vi "Initialize and Register Sessions.vi"(8 "error in":errorcluster, 11 "sequence context in":refnum<k7>) -> (0 "error out":errorcluster)   [LabVIEW 2021, in "SourceMeasureDCVoltage.lvlib"]
uses:
  SourceMeasureDCVoltage.lvlib
  <vilib>/gRPC/Generated APIs/ni/measurementlink/sessionmanagement/v1/RPC Messages/ni_measurementlink_PinMapContext.ctl
  <vilib>/Plug-In SDKs/Clients/Session Management V1/Session Reservation/Session Reservation.lvclass/Session Reservation.ctl
  FAL/Instruments/Abstract_Instrument/controls/Initialize_Info.ctl
  <vilib>/Plug-In SDKs/Clients/Session Management V1/Session Reservation/Initialize and Close Session Behavior.ctl
  <vilib>/Plug-In SDKs/Clients/Session Management V1/Session Reservation/Merge Invalid DVR Error.vi
  <vilib>/Plug-In SDKs/Clients/Session Management V1/Session Reservation/Is DVR Valid.vi
  <vilib>/Plug-In SDKs/Measurements/Helpers/Error Strings Global Internal.vi
  <vilib>/Utility/error.llb/Error Cluster From Error Code.vi
  FAL/Instruments/Abstract_Instrument/Abstract_Instrument.lvclass
  <vilib>/Plug-In SDKs/Clients/Session Management V1/Session Reservation/Session Reservation.lvclass
  <vilib>/Plug-In SDKs/TestStand/NI Pin Map TestStand.lvlib
  <vilib>/gRPC/Generated APIs/ni/measurementlink/sessionmanagement/v1/ni.measurementlink.sessionmanagement.v1.api.lvlib
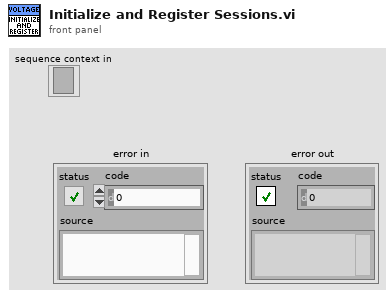
[diagram p1: front panel]
types:
  T1 = typedef "ni.measurementlink.sessionmanagement.v1.api.lvlib/ni_measurementlink_PinMapContext.ctl" = cluster{"pin_map_id":string, "sites":i32[]}
  T2 = typedef "Abstract_Instrument.lvclass/Initialize_Info.ctl" = cluster{"initialize and close session behavior":T3, "reset":bool, "optional string":string}
  T3 = typedef "NI Session Management V1 Client.lvlib/Session Reservation.lvclass/Initialize and Close Session Behavior.ctl" = enum16{"Auto", "Initialize and Close", "Attach and Detach", "Initialize and Detach", "Attach and Close"}
  T4 = typedef "ni.measurementlink.sessionmanagement.v1.api.lvlib/ni_measurementlink_sessionmanagement_v1_SessionInformation.ctl" = cluster{"session":T5, "resource_name":string, "channel_list":string, "instrument_type_id":string, "session_exists":bool, "channel_mappings":T6[]}
  T5 = typedef "ni.measurementlink.sessionmanagement.v1.api.lvlib/nidevice_grpc_Session.ctl" = cluster{"name":string}
  T6 = typedef "ni.measurementlink.sessionmanagement.v1.api.lvlib/ni_measurementlink_sessionmanagement_v1_ChannelMapping.ctl" = cluster{"pin_or_relay_name":string, "site":i32, "channel":string, "multiplexer_resource_name":string, "multiplexer_route":string}
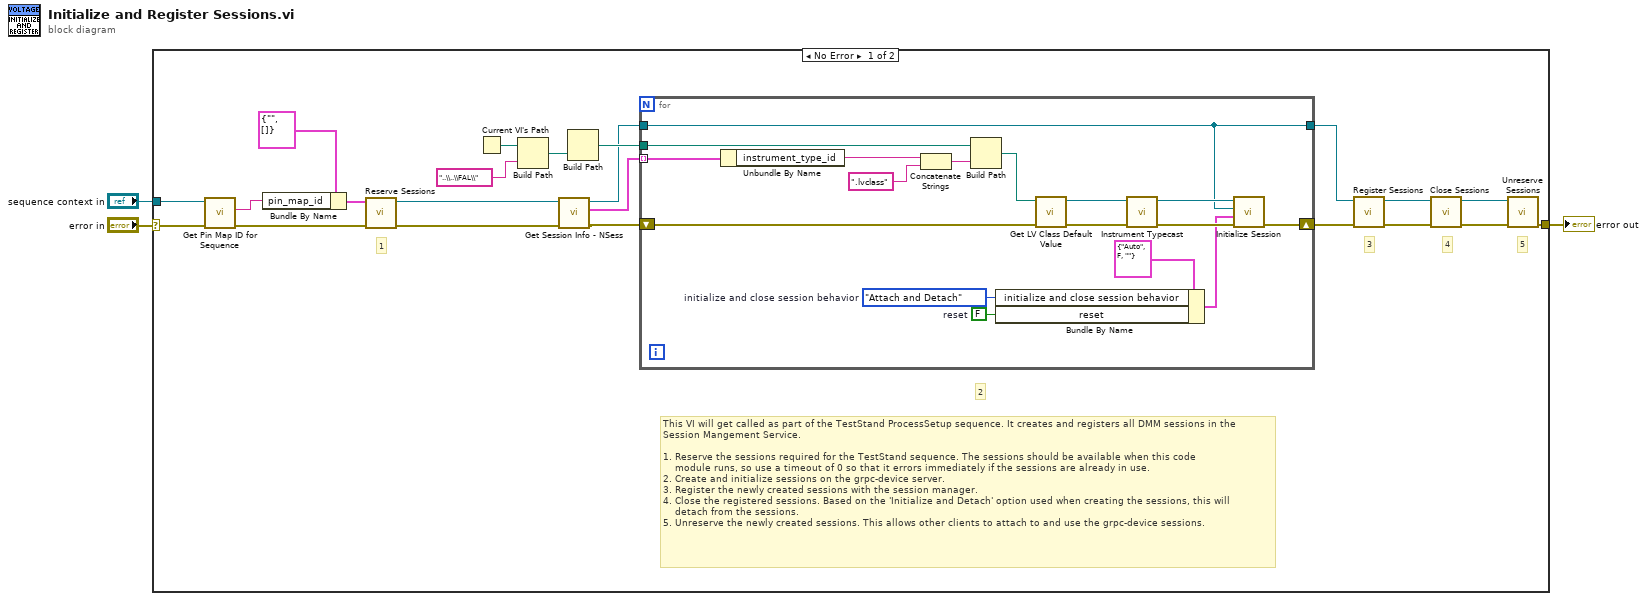
[diagram p0: block diagram]
diagram:
  n1 = case shown="No Error" "error in" {
    selector: "error in" -> [w24 w43]
    tunnel: "sequence context in" -> [w25 _]
    tunnel: [w6 w43] -> w1
    frame No Error {
      # "5"
      # "4"
      # "3"
      # "2"
      # "1"
      # "This VI will get called as part of the TestStand ProcessSetup sequence. It creates and registers all DMM sessions in the\nSession Mangement Service.\n\n1. Reserve the sessions required for the TestStand sequence. The sessions should be available when this code\n    module runs, so use a timeout of 0 so that it errors immediately if the sessions are already in use.  \n2. Create and initialize sessions on the grpc-device server.\n3. Register the newly created sessions with the session manager.\n4. Close the registered sessions. Based on the 'Initialize and Detach' option used when creating the sessions, this will\n    detach from the sessions.\n5. Unreserve the newly created sessions. This allows other clients to attach to and use the grpc-device sessions."
      n2 = call <vilib>:"Get Pin Map ID for Sequence.vi"("error in"=w24, "sequence context in"=w25) -> ("error out"=w23:errorcluster, "pin map id"=w22:string)  [unwired: 7 in, 1 out]
      n3 = Bundle By Name(cluster=T1 {"pin_map_id"="", "sites"=[]} ("pin map context"), "pin_map_id"=w22) -> (w4:T1)
      n4 = call <vilib>:"Reserve Sessions.vi"("error in"=w23, "pin map context"=w4) -> ("error out"=w12:errorcluster, "session reservation out"=w11:refnum<class "Session Reservation.lvclass">)  [unwired: 8 in]
      n5 = Current VI's Path() -> (path=w16:path)
      n6 = Build Path(base path=w16, name or relative path="..\\..\\FAL\\") -> (appended path=w15:path)
      n7 = call <vilib>:"Get Session Info - NSess .vi"("error in"=w12, "session reservation in"=w11) -> ("error out"=w19:errorcluster, "sessions info"=w18:T4[], "session reservation out"=w13:refnum<class "Session Reservation.lvclass">)  [unwired: 7 in]
      n8 = Build Path(name or relative path=w15) -> (appended path=w14:path)  [unwired: 1 in]
      n9 = for {
        shift-right: [w32] -> w8
        shift-left: w19 -> [w37]
        tunnel: w18 -> [w42] mode=indexing
        tunnel: w14 -> [w38]
        tunnel: w13 -> [w27]
        tunnel: [w27] -> w7
        w26 = Initialize_and_Close_Session_Behavior."Attach and Detach"  # initialize and close session behavior
        w28 = FALSE  # reset
        n10 = Unbundle By Name(w42) -> ("instrument_type_id"=w39:string)
        n11 = Concatenate Strings(w39, ".lvclass" ("string")) -> (w40:string)
        n12 = Build Path(base path=w38, name or relative path=w40) -> (appended path=w36:path)
        n13 = Bundle By Name(cluster=T2 {"initialize and close session behavior"=enum."Auto", "reset"=FALSE, "optional string"=""} ("Initialize_Info"), "initialize and close session behavior"=w26, "reset"=w28) -> (w29:T2)
        n14 = call <vilib>:"Get LV Class Default Value.vi"("error in (no error)"=w37, "class path"=w36) -> ("error out"=w35:errorcluster, "object"=w34:refnum<class>)  [unwired: 8 in]
        n15 = call "Instrument Typecast.vi"("error in (no error)"=w35, "pin instrument"=w34) -> ("error out"=w33:errorcluster, "instrument object"=w31:refnum<class "Abstract_Instrument.lvclass">)  [unwired: 8 in]
        n16 = call-dynamic "Initialize Session.vi"("error in (no error)"=w33, "Initialize_Info"=w29, "session reservation in"=w27, "Abstract_Instrument in"=w31) -> ("error out"=w32:errorcluster)  [unwired: 6 in, 1 out]
      }
      n17 = call <vilib>:"Register Sessions.vi"("error in"=w8, "session reservation in"=w7) -> ("error out"=w10:errorcluster, "session reservation out"=w20:refnum<class "Session Reservation.lvclass">)  [unwired: 8 in]
      n18 = call <vilib>:"Close Sessions.vi"("error in"=w10, "session reservation in"=w20) -> ("error out"=w9:errorcluster, "session reservation out"=w21:refnum<class "Session Reservation.lvclass">)  [unwired: 8 in]
      n19 = call <vilib>:"Unreserve Sessions.vi"("error in"=w9, "session reservation in"=w21) -> ("error out"=w6:errorcluster)  [unwired: 9 in]
    }
    frame Error {
    }
  }
  "error out" <- w1
